vi "PCAN_SetOneLaser.vi"(8 "Laser No":i16, 10 "Value":dbl) -> (3 "Array":u8[](array[numeric]))   [LabVIEW 2010]
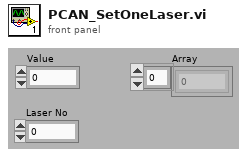
[diagram p1: front panel]
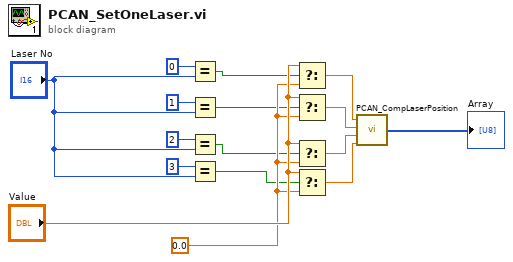
[diagram p0: block diagram]
diagram:
  w15 = 0.0 ("f")
  n1 = Equal?(x=i16 0, y="Laser No") -> (x = y?=w4:bool)
  n2 = Equal?(x=i16 1, y="Laser No") -> (x = y?=w3:bool)
  n3 = Equal?(x=i16 2, y="Laser No") -> (x = y?=w2:bool)
  n4 = Equal?(x=i16 3, y="Laser No") -> (x = y?=w1:bool)
  n5 = Select(t="Value", s=w4, f=w15) -> (s? t:f=w11:dbl)
  n6 = Select(t="Value", s=w3, f=w15) -> (s? t:f=w12:dbl)
  n7 = Select(t="Value", s=w2, f=w15) -> (s? t:f=w13:dbl)
  n8 = Select(t="Value", s=w1, f=w15) -> (s? t:f=w14:dbl)
  n9 = call "PCAN_CompLaserPosition.vi"("Laser 4"=w14, "Laser 3"=w13, "Laser 2"=w12, "Laser 1"=w11) -> ("Array"=→"Array":u8[])
